vi "Identify HSE Module.vi"(8 "error in":errorcluster, 11 "Library in":refnum<class "Library.lvclass">) -> (0 "error out":errorcluster, 3 "Library out":refnum<class "Library.lvclass">)   [LabVIEW 2020, in "Panther Dashboard.lvlib" / "Library.lvclass"]
uses:
  Library.lvclass
  LabVIEWItem/Item Type--enum.ctl
  Library.lvclass/Library.ctl
  LabVIEWItem/LabVIEWItem.lvclass/LabVIEWItem.ctl
  LabVIEWItem/Read Item Name.vi
  Read VIs MAP.vi
  Set HSE module.vi
  VI/VI.lvclass
  C:/GitClones/PantherDashboard/src/LabVIEW/Panther Dashboard/Class/LabVIEWItem/LabVIEWItem.lvclass
  LabVIEWItem/LabVIEWItem.lvclass
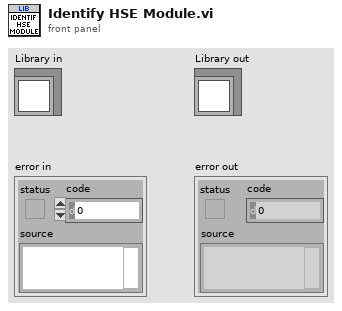
[diagram p1: front panel]
types:
  T1 = typedef "Panther Dashboard.lvlib/LabVIEWItem.lvclass/Item Type--enum.ctl" = enum16{"Requests", "Broadcasts", "Request and Wait for Reply", "Round Trip", "» Public API VIs", "» Constant VIs", "» Error VIs", "Module", "Project", "No Drag Selection"}
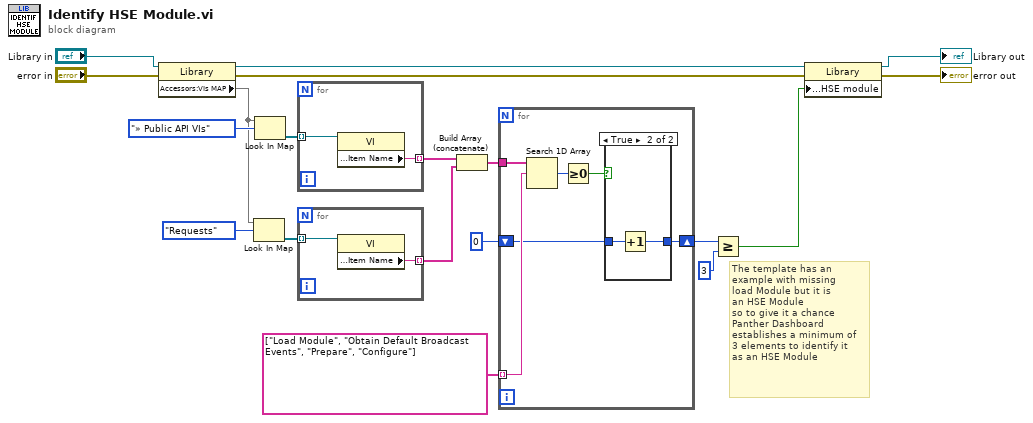
[diagram p0: block diagram]
diagram:
  # "The template has an\nexample with missing\nload Module but it is\nan HSE Module\nso to give it a chance\nPanther Dashboard\nestablishes a minimum of\n3 elements to identify it\nas an HSE Module"
  n1 = property class="Library"(reference="Library in", error in="error in") -> (reference out=w6:refnum<class "Library.lvclass">, error out=w18:errorcluster, "Accessors:VIs MAP"=w13:map{T1, refnum<class "VI.lvclass">[]})
  n2 = Look In Map(map=w13, key=Item_Type--enum."Requests") -> (value=w11:refnum<class "VI.lvclass">[])  [unwired: 1 in, 1 out]
  n3 = Look In Map(map=w13, key=Item_Type--enum."» Public API VIs") -> (value=w14:refnum<class "VI.lvclass">[])  [unwired: 1 in, 1 out]
  n4 = for {
    tunnel: w14 -> [w21] mode=indexing
    tunnel: [w20] -> w10 mode=indexing
    n5 = property class="VI"(reference=w21) -> ("Accessors:Item Name"=w20:string)  [unwired: 1 in, 2 out]
  }
  n6 = for {
    tunnel: w11 -> [w23] mode=indexing
    tunnel: [w22] -> w9 mode=indexing
    n7 = property class="VI"(reference=w23) -> ("Accessors:Item Name"=w22:string)  [unwired: 1 in, 2 out]
  }
  n8 = Build Array (concatenate)(w10, w9) -> (w8:string[])
  n9 = for {
    tunnel: w8 -> [w29]
    tunnel: string[] ["Load Module", "Obtain Default Broadcast Events", "Prepare", "Configure"] -> [w28] mode=indexing
    shift-right: [w25] -> w3
    shift-left: 0 -> [w24]
    n10 = Search 1D Array(1D array=w29, element=w28) -> (index of element=w27:i32)  [unwired: 1 in]
    n11 = Greater Or Equal To 0?(x=w27) -> (x >= 0?=w26:bool)
    n12 = case shown="True" w26 {
      tunnel: [w30 w32] -> w25
      tunnel: w24 -> [w30 w31]
      frame False {
      }
      frame True {
        n13 = Increment(x=w31) -> (x+1=w32:i32)
      }
    }
  }
  n14 = Greater Or Equal?(x=w3, y=3) -> (x >= y?=w2:bool)
  n15 = property class="Library"(reference=w6, error in=w18, "Accessors:HSE module"=w2) -> (reference out=→"Library out":refnum<class "Library.lvclass">, error out=→"error out":errorcluster)
